vi "Fan Speed Acquisition.vi"(6 "Control Index":i32, 8 "error in (no error)":errorcluster, 9 "channel":T1, 10 "Stream in":refnum<class "Stream.lvclass">, 11 "DAQmx Task In":refnum<k21>) -> (0 "error out":errorcluster, 3 "DAQmx Task Out":refnum<k21>)   [LabVIEW 2020]
uses:
  <extravilib>/ChannelInstances/Tag-bool/))Channel.ctl
  submodules/nominal-streaming-labview-ffi/lv_src/Stream/Stream.lvclass
  <vilib>/DAQmx/read.llb/DAQmx Read (Counter DBL 1Chan 1Samp).vi
  <extravilib>/ChannelInstances/Tag-bool/Read With Abort.vi
  <extravilib>/ChannelInstances/Tag-bool/EndpointRead.vi
  <vilib>/DAQmx/miscellaneous.llb/DAQmx Fill In Error Info.vi
  <vilib>/ptbypt/NI_PtbyPt.lvlib
  <extravilib>/ChannelInstances/Tag-bool.lvlib
  submodules/nominal-streaming-labview-ffi/lv_src/Channel/Channel.lvclass
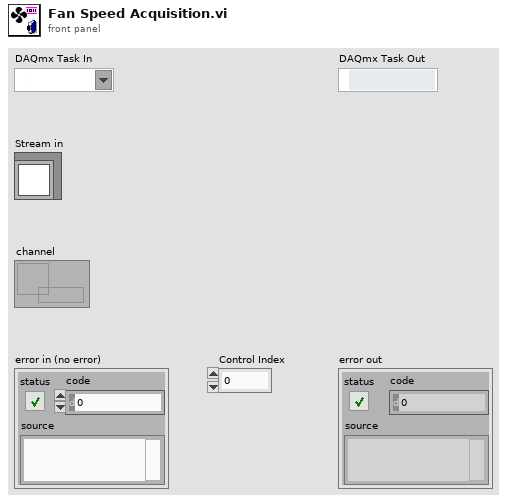
[diagram p1: front panel]
types:
  T1 = typedef "Tag-bool.lvlib/))Channel.ctl" = refnum<queue>
  T2 = cluster{"seconds since 1Jan1904":timestamp, "x":dbl}
  T3 = cluster{"seconds since 1Jan1904":timestamp, "x":dbl}[]
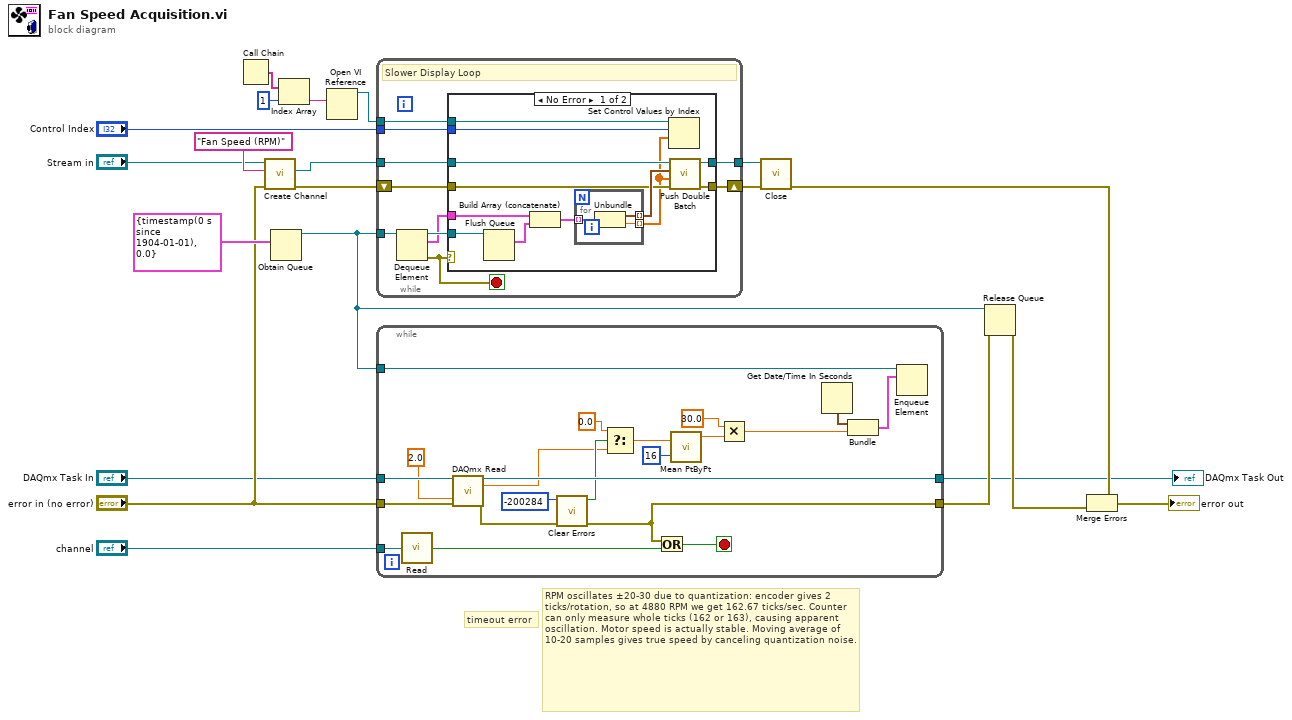
[diagram p0: block diagram]
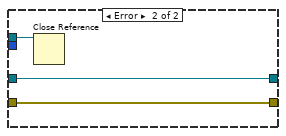
[diagram p2: hidden frame]
diagram:
  # "timeout error"
  # "RPM oscillates ±20-30 due to quantization: encoder gives 2 ticks/rotation, so at 4880 RPM we get 162.67 ticks/sec. Counter can only measure whole ticks (162 or 163), causing apparent oscillation. Motor speed is actually stable. Moving average of 10-20 samples gives true speed by canceling quantization noise."
  n1 = Call Chain() -> (call chain=w5:string[])
  n2 = call "Create Channel.vi"("error in (no error)"="error in (no error)", "Channel Name"="Fan Speed (RPM)", "Nominal Streaming in"="Stream in") -> ("error out"=w14:errorcluster, "Channel"=w13:refnum<class "Channel.lvclass">)  [unwired: 6 in, 1 out]
  n3 = Obtain Queue(element data type=T2 {"seconds since 1Jan1904"=timestamp(0 s since 1904-01-01), "x"=0.0} ("output cluster")) -> (queue out=w19:refnum<queue>)  [unwired: 4 in, 2 out]
  n4 = Index Array(array=w5, index=1) -> (element=w3:string)
  n5 = Open VI Reference(vi path=w3) -> (vi reference=w2:refnum<vi>)  [unwired: 5 in, 1 out]
  n6 = while {
    tunnel: [w27] -> w11
    tunnel: w13 -> [w28]
    shift-right: [w26] -> w15
    shift-left: w14 -> [w25]
    tunnel: w19 -> [w31]
    tunnel: w2 -> [w23]
    tunnel: "Control Index" -> [w22]
    stop <- w24 stop-if-true
    # "Slower Display Loop"
    n7 = Dequeue Element(queue=w31) -> (queue out=w30:refnum<queue>, element=w29:T2, error out=w24:errorcluster)  [unwired: 2 in, 1 out]
    n8 = case shown="No Error" w24 {
      tunnel: w30 -> [w43 _]
      tunnel: w29 -> [w41 _]
      tunnel: w28 -> [w36 w49]
      tunnel: [w33 w49] -> w27
      tunnel: [w32 w48] -> w26
      tunnel: w25 -> [w35 w48]
      tunnel: w23 -> [w39 w47]
      tunnel: w22 -> [w38 _]
      frame No Error {
        n9 = Flush Queue(queue=w43) -> (remaining elements=w42:T3)  [unwired: 1 in, 2 out]
        n10 = Build Array (concatenate)(w41, w42) -> (w40:T3)
        n11 = for {
          tunnel: w40 -> [w46] mode=indexing
          tunnel: [w45] -> w37 mode=indexing
          tunnel: [w44] -> w34 mode=indexing
          n12 = Unbundle(w46) -> ("seconds since 1Jan1904"=w45:timestamp, "x"=w44:dbl)
        }
        n13 = Set Control Values by Index(0:w39, 1:w38, 2:w34) -> ()  [unwired: 1 in, 1 out]
        n14 = call "Push Double Batch.vi"("error in (no error)"=w35, "Values"=w34, "Timestamps"=w37, "Channel in"=w36) -> ("error out"=w32:errorcluster, "Channel out"=w33:refnum<class "Channel.lvclass">)  [unwired: 6 in]
      }
      frame Error {
        n15 = Close Reference(reference=w47) -> ()  [unwired: 1 in, 1 out]
      }
    }
  }
  n16 = while {
    tunnel: "DAQmx Task In" -> [w70]
    tunnel: "error in (no error)" -> [w69]
    tunnel: [w62] -> w20
    tunnel: [w67] -> w7
    tunnel: "channel" -> [w55]
    tunnel: w19 -> [w52]
    stop <- w68 stop-if-true
    n17 = call <extravilib>:"Read.vi"("channel"=w55) -> ("element"=w54:bool)  [unwired: 1 in, 1 out]
    n18 = call-poly <vilib>:"DAQmx Read.vi"("task/channels in"=w70, "timeout"=2.0, "error in"=w69) -> ("task out"=w67:refnum<k21>, "data"=w59:dbl, "error out"=w63:errorcluster)  [unwired: 10 in]
    n19 = call <vilib>:"Clear Errors.vi"("error in (no error)"=w63, "specific error code to clear (0: all)"=-200284) -> ("error out"=w62:errorcluster, "specific error cleared?"=w60:bool)  [unwired: 4 in]
    n20 = Select(t=0.0, s=w60, f=w59) -> (s? t:f=w57:dbl)
    n21 = Or(x=w62, y=w54) -> (x .or. y?=w68:bool)
    n22 = call <vilib>:"Mean PtByPt.vi"("x"=w57, "sample length"=16) -> ("mean"=w56:dbl)  [unwired: 2 in, 1 out]
    n23 = Multiply(x=30.0 ("y"), y=w56) -> (x*y=w50:dbl)
    n24 = Get Date/Time In Seconds() -> (seconds since 1Jan1904=w51:timestamp)
    n25 = Bundle("seconds since 1Jan1904"=w51, w50) -> (w53:cluster{"seconds since 1Jan1904":timestamp, dbl})  [unwired: 1 in]
    n26 = Enqueue Element(queue=w52, element=w53) -> ()  [unwired: 2 in, 3 out]
  }
  "DAQmx Task Out" <- w7
  n27 = call "Close.vi"("error in (no error)"=w15, "Channel in"=w11) -> ("error out"=w10:errorcluster)  [unwired: 9 in]
  n28 = Release Queue(queue=w19, error in (no error)=w20) -> (error out=w9:errorcluster)  [unwired: 1 in, 2 out]
  n29 = Merge Errors(w10, w9) -> (→"error out":errorcluster)
